vi "Target.vi"() -> ()   [LabVIEW 2018]
uses:
  <vilib>/rvi/Emulation/niFpgaGetClockAttributes.vi
  <vilib>/rvi/Emulation/niFpgaSctlEmulationGetInTimedLoop.vi
  <vilib>/rvi/Emulation/niFpgaEmulationReportErrorSimple.vi
  <vilib>/rvi/eio/common/nirviEmuTemplateMethod_errors.vi
  <vilib>/rvi/Emulation/niFpgaCriticalErrorInLSC.vi
  <vilib>/eio/EIONode/EIONode.xnode
panel:
  out "Connector0/AI7":i16
  out "Connector0/AI6":i16
  in  "Connector0/AO2":i16
  in  "Connector0/AO3":i16
  in  "Connector0/AO1":i16
  in  "Connector0/AO0":i16
  out "Connector0/AI5":i16
  out "Connector0/AI4":i16
  out "Connector0/AI3":i16
  out "Connector0/AI2":i16
  out "Connector0/AI1":i16
  out "Connector0/AI0":i16
  in  "Стоп":bool
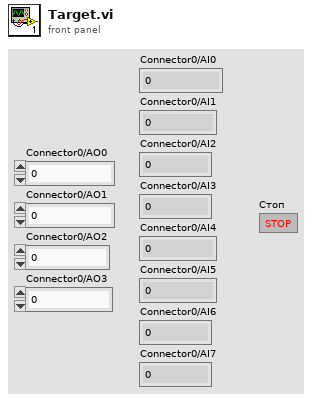
[diagram p1: front panel]
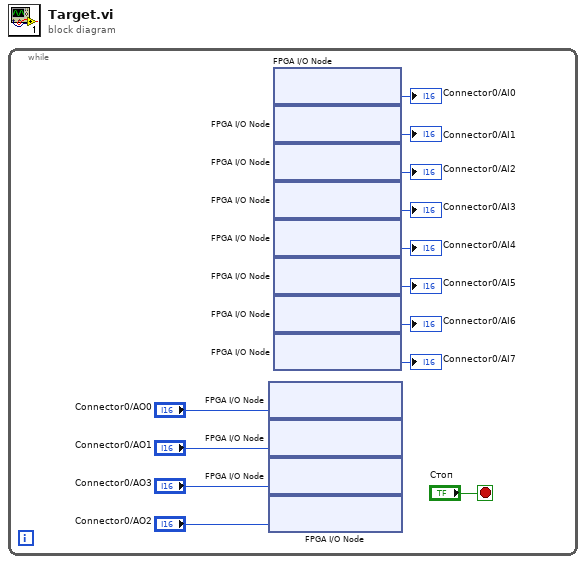
[diagram p0: block diagram]
diagram:
  n1 = while {
    stop <- "Стоп" stop-if-true
    n2 = xnode "FPGA I/O Node"("Connector0/AO0"="Connector0/AO0") -> ()  [unwired: 1 in, 1 out]
    n3 = xnode "FPGA I/O Node"("Connector0/AO1"="Connector0/AO1") -> ()  [unwired: 1 in, 1 out]
    n4 = xnode "FPGA I/O Node"("Connector0/AO3"="Connector0/AO3") -> ()  [unwired: 1 in, 1 out]
    n5 = xnode "FPGA I/O Node"("Connector0/AO2"="Connector0/AO2") -> ()  [unwired: 1 in, 1 out]
    n6 = xnode "FPGA I/O Node"() -> ("Connector0/AI0"=→"Connector0/AI0":i16)  [unwired: 1 in, 1 out]
    n7 = xnode "FPGA I/O Node"() -> ("Connector0/AI1"=→"Connector0/AI1":i16)  [unwired: 1 in, 1 out]
    n8 = xnode "FPGA I/O Node"() -> ("Connector0/AI2"=→"Connector0/AI2":i16)  [unwired: 1 in, 1 out]
    n9 = xnode "FPGA I/O Node"() -> ("Connector0/AI3"=→"Connector0/AI3":i16)  [unwired: 1 in, 1 out]
    n10 = xnode "FPGA I/O Node"() -> ("Connector0/AI4"=→"Connector0/AI4":i16)  [unwired: 1 in, 1 out]
    n11 = xnode "FPGA I/O Node"() -> ("Connector0/AI5"=→"Connector0/AI5":i16)  [unwired: 1 in, 1 out]
    n12 = xnode "FPGA I/O Node"() -> ("Connector0/AI6"=→"Connector0/AI6":i16)  [unwired: 1 in, 1 out]
    n13 = xnode "FPGA I/O Node"() -> ("Connector0/AI7"=→"Connector0/AI7":i16)  [unwired: 1 in, 1 out]
  }
